vi "LakeShore370 Control Panel.vi"(8 "error in (no error)":errorcluster, 11 "Class":refnum<class "LakeShore370_device.lvclass">) -> (0 "error out":errorcluster, 3 "LakeShore370 out":refnum<class "LakeShore370_device.lvclass">)   [LabVIEW 2015, in "LakeShore370_device.lvclass"]
uses:
  LakeShore370_device.lvclass
  LakeSore370 Front Panel Data.ctl
  LakeShore370 Heater Ranges.ctl
  Neocera/Neocera Set Point Aproach.ctl
panel:
  in  "Data":T1={"Channels to scan"=[], "Scan settling, s"=10.0, "Read temperature"=FALSE, "Set point"=0.0, "Heater range"=enum."Off", "Approach"=enum."Instant", "Ramp rate, K/min"=1.0, "Read heater"=FALSE}
  # "Scanner"
  # "Temperature Control"
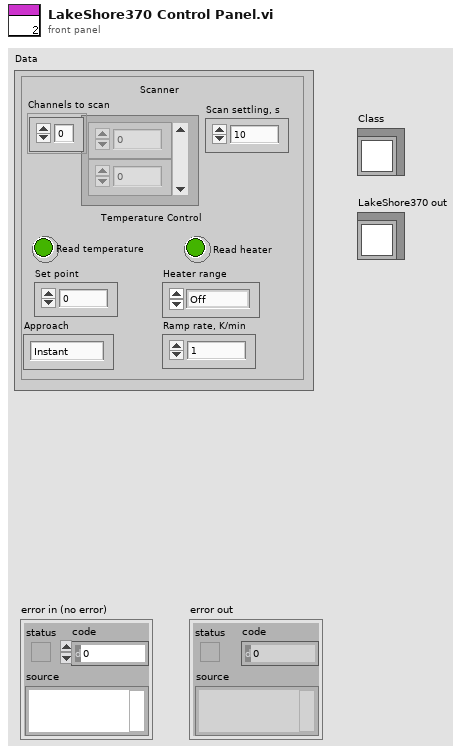
[diagram p1: front panel]
types:
  T1 = typedef "LakeSore370 Front Panel Data.ctl" = cluster{"Channels to scan":i32[], "Scan settling, s":dbl, "Read temperature":bool, "Set point":dbl, "Heater range":T2, "Approach":T3, "Ramp rate, K/min":dbl, "Read heater":bool}
  T2 = typedef "LakeShore370 Heater Ranges.ctl" = enum16{"Off", "31.6uA", "100uA", "316uA", "1mA", "3.16uA", "10mA", "31.6mA", "100mA"}
  T3 = typedef "Neocera Set Point Aproach.ctl" = enum16{"Instant", "Ramp"}
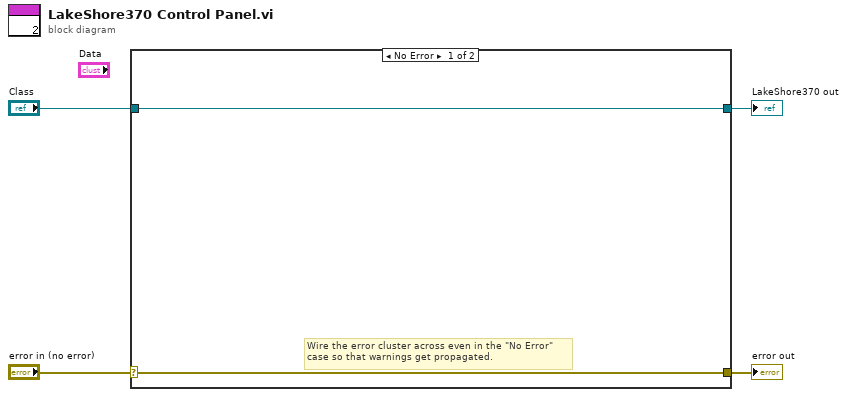
[diagram p0: block diagram]
diagram:
  n1 = case shown="No Error" "error in (no error)" {
    selector: "error in (no error)" -> [w5 w8]
    tunnel: [w5 w8] -> w3
    tunnel: [w6 w7] -> w1
    tunnel: "Class" -> [w6 w7]
    frame No Error {
      # "Wire the error cluster across even in the \"No Error\"\ncase so that warnings get propagated."
    }
    frame Error {
    }
  }
  "error out" <- w3
  "LakeShore370 out" <- w1
